vi "R&S Set RF.vi"() -> (0 "Error":bool)   [LabVIEW 2009]
doc: "This device configures the Rohde & Schwarz RF Generator for use. The central frequency, modulation, RF power, and GPIB address are taken from the QCA Global."
uses:
  QCA Global.vi
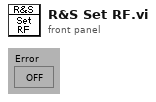
[diagram p1: front panel]
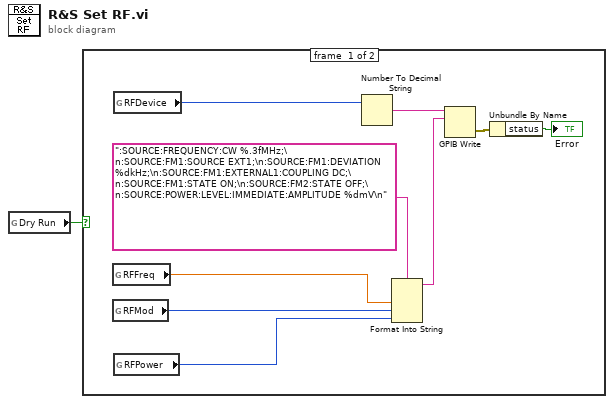
[diagram p0: block diagram]
diagram:
  n1 = global read "QCA Global.vi" "Dry Run"() -> (w1:bool)
  n2 = case shown="False" w1 {
    frame #0 {
      n3 = global read "QCA Global.vi" "RFFreq"() -> (w6:dbl)
      n4 = global read "QCA Global.vi" "RFMod"() -> (w3:i32)
      n5 = global read "QCA Global.vi" "RFDevice"() -> (w5:i32)
      n6 = global read "QCA Global.vi" "RFPower"() -> (w2:i32)
      n7 = Number To Decimal String(number=w5) -> (decimal integer string=w4:string)  [unwired: 1 in]
      n8 = Format Into String(format string=":SOURCE:FREQUENCY:CW %.3fMHz;\n:SOURCE:FM1:SOURCE EXT1;\n:SOURCE:FM1:DEVIATION %dkHz;\n:SOURCE:FM1:EXTERNAL1:COUPLING DC;\n:SOURCE:FM1:STATE ON;\n:SOURCE:FM2:STATE OFF;\n:SOURCE:POWER:LEVEL:IMMEDIATE:AMPLITUDE %dmV\n", w6, w3, w2) -> (resulting string=w9:string)  [unwired: 2 in, 1 out]
      n9 = GPIB Write(0:w4, 1:w9) -> (6:w8:errorcluster)  [unwired: 3 in, 1 out]
      n10 = Unbundle By Name(w8) -> ("status"=→"Error":bool)
    }
    frame #1 {
    }
  }
